vi "config.vi"(4 "feedback":bool, 5 "dragc":dbl, 6 "sizeofimgz":i32, 7 "sizeofimgx":i32, 9 "scopez":i32, 10 "scopex":i32, 11 "ypos":dbl) -> ()   [LabVIEW 2017, in "HapticSTM.lvlib"]
doc: "extern \"C\" __declspec(dllexport) void config(double ypos, int scopex, int scopez, int sizeofimgx, int sizeofimgz, double dragc, bool feedback);"
uses:
  HapticSTM.lvlib
  <userlib>/HapticSTM/HapticSTM.dll
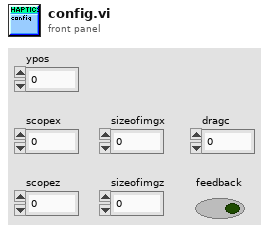
[diagram p1: front panel]
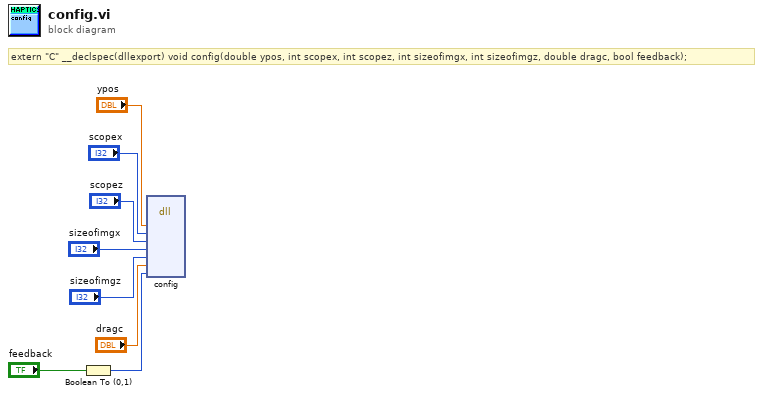
[diagram p0: block diagram]
diagram:
  # "extern \"C\" __declspec(dllexport) void config(double ypos, int scopex, int scopez, int sizeofimgx, int sizeofimgz, double dragc, bool feedback);"
  n1 = Boolean To (0,1)(Boolean="feedback") -> (0, 1=w1:i16)
  n2 = dll-call lib="C:/Program Files/National Instruments/LabVIEW 2019/user.lib/HapticSTM/HapticSTM.*" fn="config"("ypos"="ypos", "scopex"="scopex", "scopez"="scopez", "sizeofimgx"="sizeofimgx", "sizeofimgz"="sizeofimgz", "dragc"="dragc", "feedback"=w1) -> ()  [unwired: 11 in, 2 out]
